vi "solar_qtimer Obtain.vi"(6 "Suppress Errors? (T)":bool=TRUE, 8 "error in (no error)":errorcluster, 9 "Create if not found? (T)":bool=TRUE, 11 "Interface":string) -> (0 "error out":errorcluster, 3 "QTimer Refnum":T1)   [LabVIEW 2018]
doc: "This obtains a reference to the QTimer interface that controls all QTimers within a SOLAR application."
uses:
  solar_qtimer_ctl QTimer.ctl
  solar_qtimer_ctl SEQ.ctl
  solar_qtimer_ctl QTimer Settings.ctl
  solar_qtimer_ctl Refnum.ctl
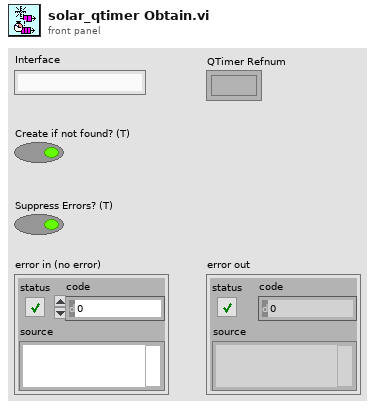
[diagram p1: front panel]
types:
  T1 = typedef "solar_qtimer_ctl Refnum.ctl" = refnum<k1>
  T2 = typedef "solar_qtimer_ctl SEQ.ctl" = cluster{"QTimers":T3[]}
  T3 = typedef "solar_qtimer_ctl QTimer.ctl" = cluster{"Settings":T4, "Queue":refnum<queue>, "QTimerQ":refnum<queue>, "VI Refnum":refnum<vi>}
  T4 = typedef "solar_qtimer_ctl QTimer Settings.ctl" = cluster{"QTimer":string, "Delay":i32, "Start":bool, "EnQ_Type":enum8{"Normal", "Priority", "IgnoreIfExists"}, "Messages":cluster{"MSG":string, "DATA":variant}[]}
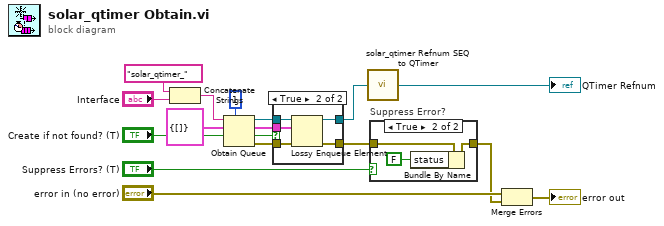
[diagram p0: block diagram]
diagram:
  w8 = T2 {"QTimers"=[]} ("QTimers")
  n1 = Concatenate Strings("solar_qtimer_" ("string"), "Interface") -> (w14:string)
  n2 = Obtain Queue(max queue size (-1, unlimited)=1, name (unnamed)=w14, element data type=w8, create if not found? (T)="Create if not found? (T)") -> (queue out=w11:refnum<queue>, created new?=w10:bool, error out=w9:errorcluster)  [unwired: 1 in]
  n3 = case shown="True" w10 {
    tunnel: w11 -> [w18 w23]
    tunnel: w8 -> [_ w22]
    tunnel: w9 -> [w17 w21]
    tunnel: [w18 w20] -> w7
    tunnel: [w17 w19] -> w2
    frame False {
    }
    frame True {
      n4 = Lossy Enqueue Element(queue=w23, element=w22, error in (no error)=w21) -> (queue out=w20:refnum<queue>, error out=w19:errorcluster)  [unwired: 2 out]
    }
  }
  n5 = call "solar_qtimer Refnum SEQ to QTimer.vi"("QTimers SEQ"=w7) -> ("QTimer Refnum"=→"QTimer Refnum":T1)
  n6 = case "Suppress Error?" shown="True" "Suppress Errors? (T)" {
    tunnel: w2 -> [w24 w27]
    tunnel: [w24 w26] -> w1
    frame False {
    }
    frame True {
      n7 = Bundle By Name(cluster=w27, "status"=FALSE) -> (w26:errorcluster)
    }
  }
  n8 = Merge Errors("error in (no error)", w1) -> (→"error out":errorcluster)
